vi "Generate Path.vi"(0 "path":T2[](array[typedef]), 5 "max_velocity":dbl, 7 "max_acceleration":dbl, 9 "max_jerk":dbl, 11 "error in":errorcluster, 12 "dt (.001)":dbl=0.001, 13 "sample_count (100000)":i32=100000) -> (4 "Segments":T1[](array[typedef]), 15 "error out":errorcluster)   [LabVIEW 2017, in "Pathfinder.lvlib"]
uses:
  Pathfinder.lvlib
  Waypoint.ctl
  Segment.ctl
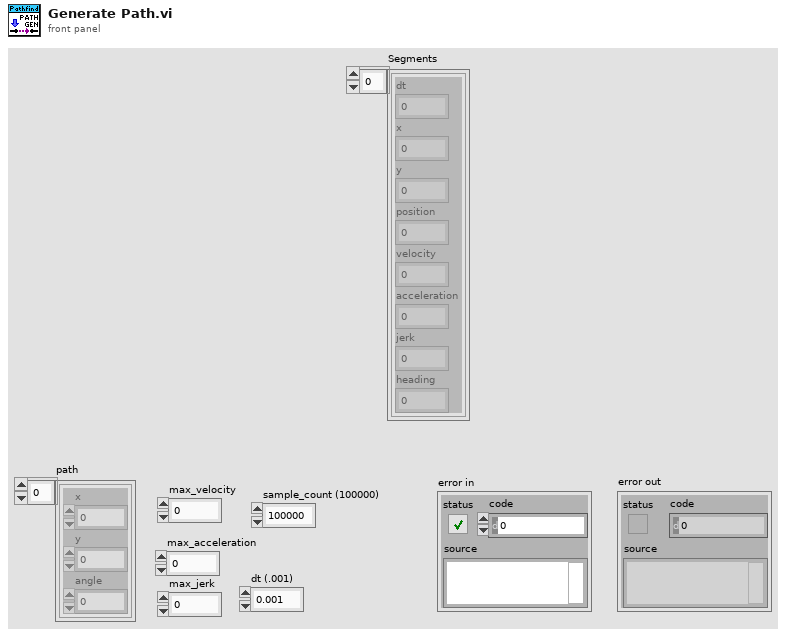
[diagram p1: front panel]
types:
  T1 = typedef "Pathfinder.lvlib/Segment.ctl" = cluster{"dt":dbl, "x":dbl, "y":dbl, "position":dbl, "velocity":dbl, "acceleration":dbl, "jerk":dbl, "heading":dbl}
  T2 = typedef "Pathfinder.lvlib/Waypoint.ctl" = cluster{"x":dbl, "y":dbl, "angle":dbl}
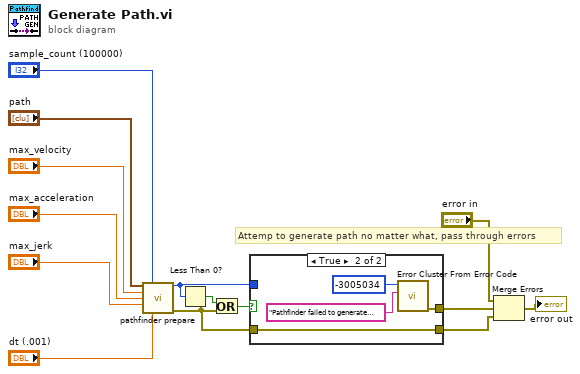
[diagram p0: block diagram]
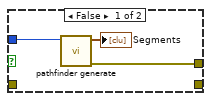
[diagram p2: hidden frame]
diagram:
  # "Attemp to generate path no matter what, pass through errors"
  n1 = call "pathfinder prepare.vi"("path"="path", "sample_count"="sample_count (100000)", "max_velocity"="max_velocity", "max_acceleration"="max_acceleration", "max_jerk"="max_jerk", "dt"="dt (.001)") -> ("function return"=w9:i32, "error out"=w2:errorcluster)  [unwired: 8 in]
  n2 = Less Than 0?(x=w9) -> (x < 0?=w14:bool)
  n3 = Or(x=w14, y=w2) -> (x .or. y?=w13:bool)
  n4 = case shown="True" w13 {
    tunnel: [w17 w21] -> w10
    tunnel: w9 -> [w16 _]
    tunnel: w2 -> [_ w18]
    tunnel: [_ w18] -> w1
    frame False {
      n5 = call "pathfinder generate.vi"("trajectory length"=w16) -> ("error out"=w17:errorcluster, "Segments"=→"Segments":T1[])  [unwired: 9 in]
    }
    frame True {
      n6 = call <vilib>:"Error Cluster From Error Code.vi"("error message (\"\")"="Pathfinder failed to generate trajectory" ("error message (\"\")"), "error code (0)"=-3005034) -> ("error out"=w21:errorcluster)  [unwired: 7 in]
    }
  }
  n7 = Merge Errors("error in", w10, w1) -> (→"error out":errorcluster)
